vi "Device ON_OFF & Wifi_Connection.vi"(8 "error in":errorcluster) -> (0 "error out":errorcluster, 2 "DUT COM port":bool, 3 "Wifi Connected":bool, 5 "Device Not respond":bool)   [LabVIEW 2019]
panel:
  out "match substring":string
  out "standard output":string
  out "standard error":string
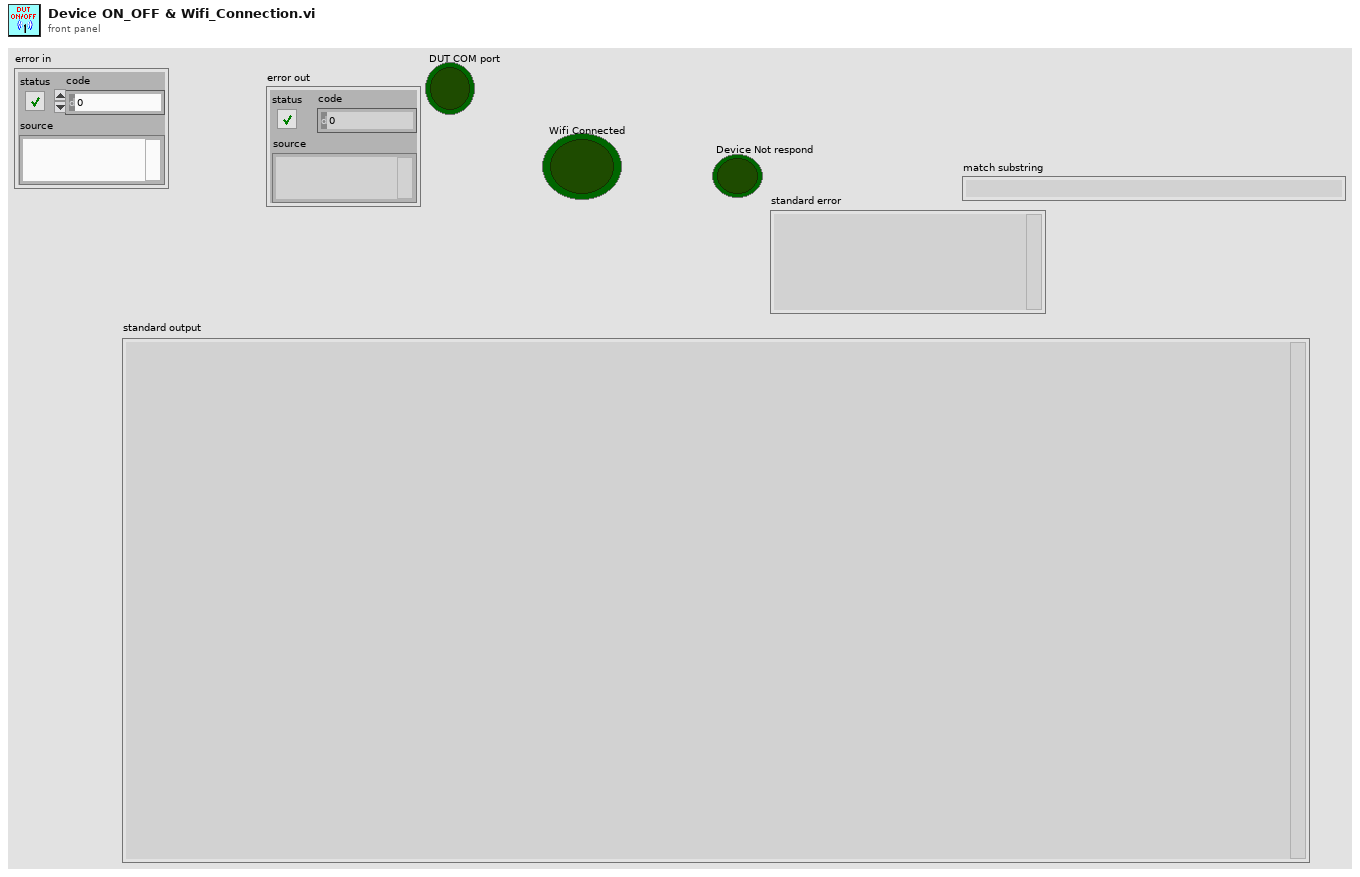
[diagram p1: front panel]
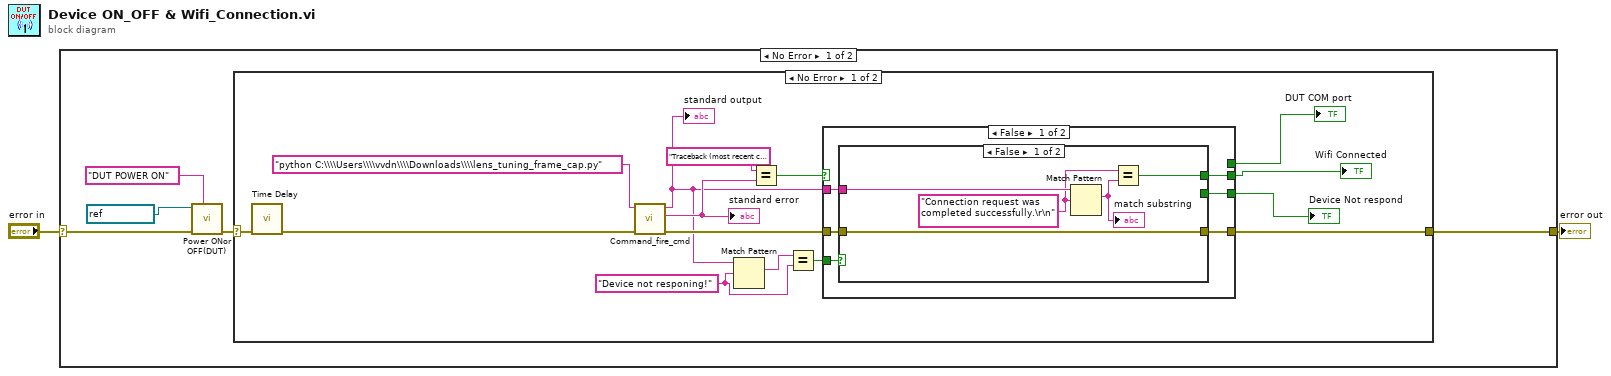
[diagram p0: block diagram]
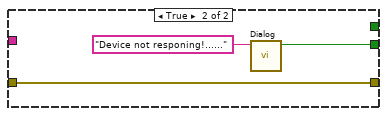
[diagram p2: hidden frame]
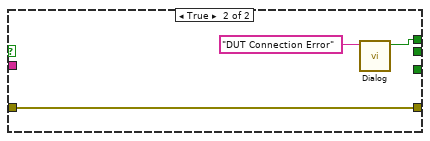
[diagram p3: hidden frame]
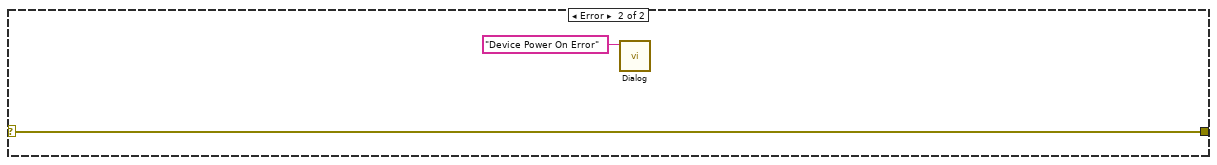
[diagram p4: hidden frame]
diagram:
  n1 = case shown="No Error" "error in" {
    selector: "error in" -> [w4 w42]
    tunnel: [w7 w42] -> w2
    frame No Error {
      n2 = call "Power ONor OFF(DUT).vi"("String"="DUT POWER ON", "error in (no error)"=w4, "VISA resource name"=refnum<visa-resource-name> "COM11") -> ("error out"=w3:errorcluster)  [unwired: 8 in]
      n3 = case shown="No Error" w3 {
        selector: w3 -> [w21 w40]
        tunnel: [w22 w40] -> w7
        frame No Error {
          w11 = "Device not responing!"
          n4 = call "Time Delay"("error in (no error)"=w21) -> ("error out"=w19:errorcluster)  [unwired: 10 in]
          n5 = call "Command_fire_cmd.vi"("error in"=w19, "command line"="python C:\\\\Users\\\\vvdn\\\\Downloads\\\\lens_tuning_frame_cap.py") -> ("error out"=w18:errorcluster, "standard error"=w14:string, "standard output"=w8:string)  [unwired: 5 in]
          "standard error" <- w14
          "standard output" <- w8
          n6 = Match Pattern(string=w8, regular expression=w11) -> (match substring=w12:string)  [unwired: 1 in, 3 out]
          n7 = Equal?(x="Traceback (most recent call last):\r\n  File \"C:\\Users\\vvdn\\Downloads\\lens_tuning_frame_cap.py\", line 1067, in <module>\r\n    run()\r\n  File \"C:\\Users\\vvdn\\Downloads\\lens_tuning_frame_cap.py\", line 749, in run\r\n    new_thread()\r\n  File \"C:\\Users\\vvdn\\Downloads\\lens_tuning_frame_cap.py\", line 767, in new_thread\r\n    print(DUT_port.readlines())\r\nAttributeError: 'NoneType' object has no attribute 'readlines'\r\n" ("standard error 2"), y=w14) -> (x = y?=w17:bool)
          n8 = Equal?(x=w12, y=w11) -> (x = y?=w13:bool)
          n9 = case shown="False" w17 {
            tunnel: [w25 w39] -> w22
            tunnel: [w27 _] -> w9
            tunnel: w18 -> [w26 w39]
            tunnel: [_ w37] -> w15
            tunnel: w8 -> [w28 _]
            tunnel: w13 -> [w24 _]
            tunnel: [w23 _] -> w10
            frame False {
              n10 = case shown="False" w24 {
                tunnel: w28 -> [w33 _]
                tunnel: [w30 _] -> w27
                tunnel: w26 -> [w29 w36]
                tunnel: [w29 w36] -> w25
                tunnel: [_ w34] -> w23
                frame False {
                  w31 = "Connection request was completed successfully.\r\n" ("standard output 3")
                  n11 = Match Pattern(string=w33, regular expression=w31) -> (match substring=w32:string)  [unwired: 1 in, 3 out]
                  "match substring" <- w32
                  n12 = Equal?(x=w31, y=w32) -> (x = y?=w30:bool)
                }
                frame True {
                  n13 = call "Dialog.vi"("Status"="Device not responing!......") -> ("Cancelled?"=w34:bool)  [unwired: 10 in]
                }
              }
            }
            frame True {
              n14 = call "Dialog.vi"("Status"="DUT Connection Error") -> ("Cancelled?"=w37:bool)  [unwired: 10 in]
            }
          }
          "DUT COM port" <- w15
          "Device Not respond" <- w10
          "Wifi Connected" <- w9
        }
        frame Error {
          n15 = call "Dialog.vi"("Status"="Device Power On Error") -> ()  [unwired: 10 in, 1 out]
        }
      }
    }
    frame Error {
    }
  }
  "error out" <- w2
